vi "Set_Hi-Tec_client.vi"(4 "Gas Line Name":T1, 5 "Row No":i32=1, 6 "Strength (% by volume)":dbl format="%.2f", 7 "Carrier_2 Q (l/min)":dbl=20.0 format="%.2f", 8 "Carrier_1 Q (l/min)":dbl=20.0 format="%.2f", 9 "Mode":enum16{"Control Hi-Tec", "Check Hi-Tec Demands"}(ring)) -> (0 "error out":errorcluster, 1 "Flowrates (kg/min)":dbl[](array[numeric]) format="%.4f")   [LabVIEW 2022 SP3]
doc: "This is an example of using features of the VI Server as a client. It shows how you might browse from one or more applications that may be exporting data from one or more data stations. \n\nThe example shows how to query a server for its list of exported VIs, how to get references to the VIs, and how call them with the Call By Reference function."
uses:
  Anemometry/Anemometry Sub Vis/Controls/GMU Gas Line Name.ctl
  Anemometry/Anemometry Sub Vis/Globals/Preference_global.vi
panel:
  out "Iterations":i32
  in  "Server type":refnum<vi>
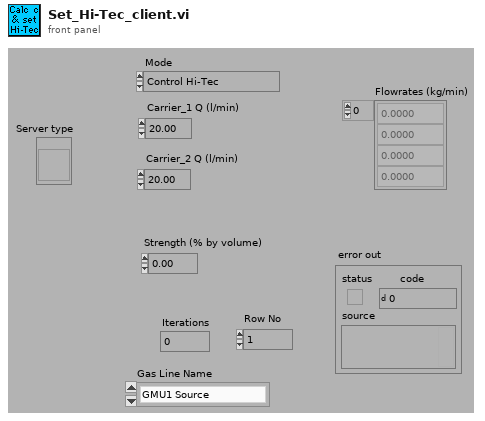
[diagram p1: front panel]
types:
  T1 = typedef "GMU Gas Line Name.ctl" = enum16{"GMU1 Source", "GMU2 Source", "GMU2 Calib", "CPP GRC-A", "CPP GRC-B"}
  T2 = typedef "Server_Comms.ctl" = enum16{"Do Not Link To Server", "Server Link Healthy"}
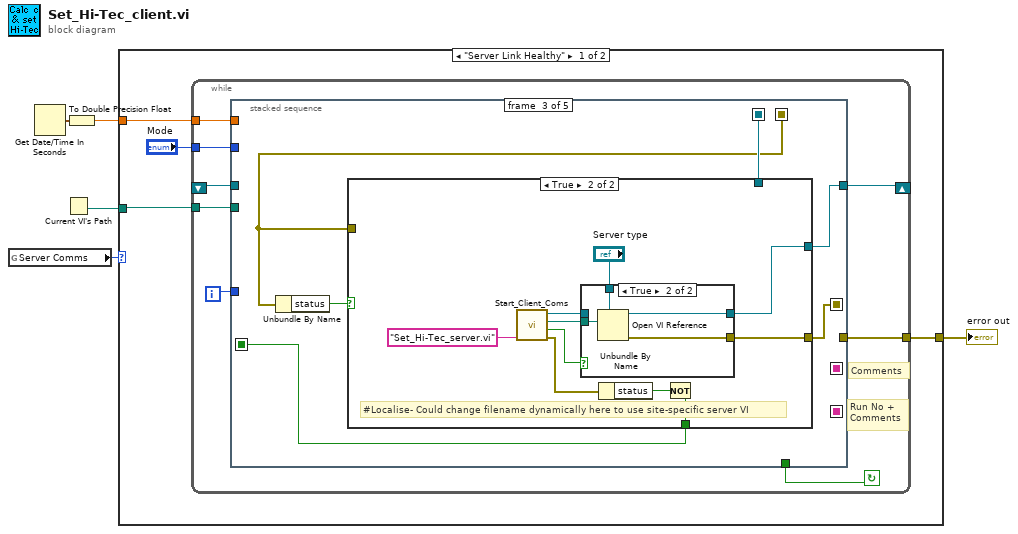
[diagram p0: block diagram]
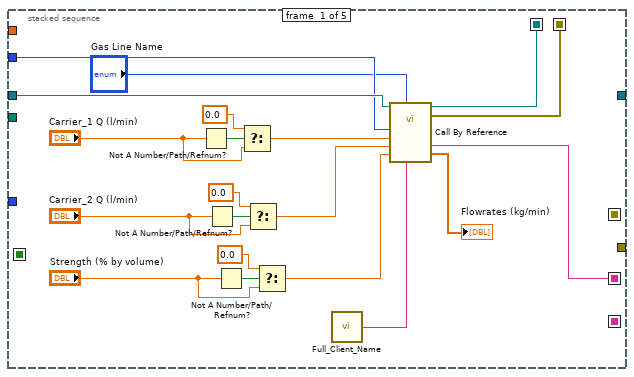
[diagram p2: hidden frame]
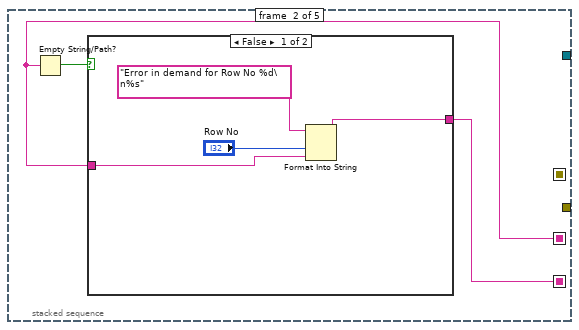
[diagram p3: hidden frame]
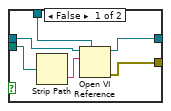
[diagram p6: hidden frame]
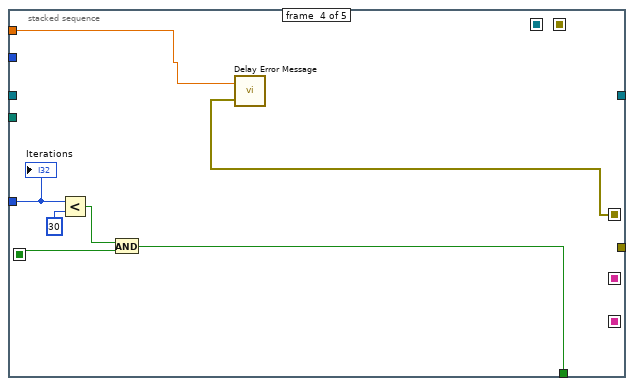
[diagram p7: hidden frame]
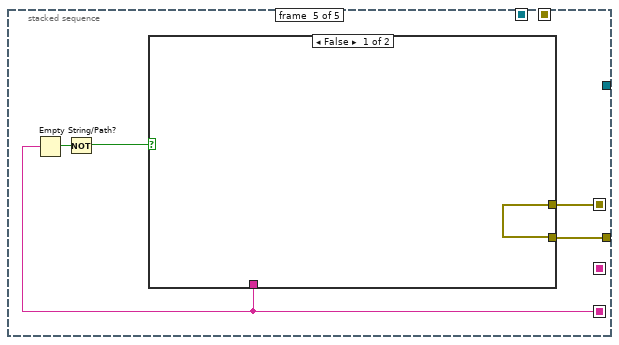
[diagram p8: hidden frame]
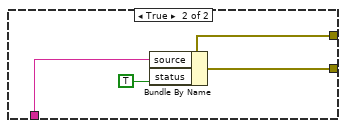
[diagram p9: hidden frame]
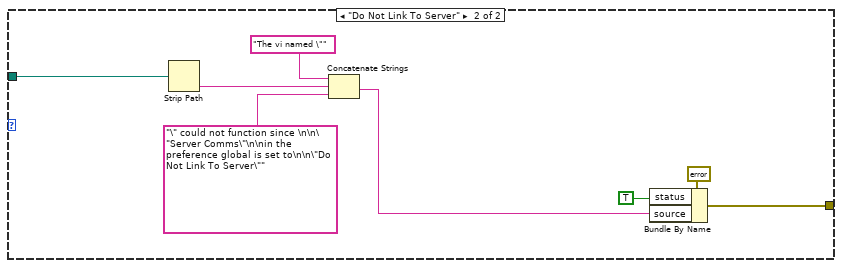
[diagram p10: hidden frame]
diagram:
  n1 = global read "Preference_global.vi" "Server Comms"() -> (w5:T2)
  n2 = Get Date/Time In Seconds() -> (seconds since 1Jan1904=w2:timestamp)
  n3 = Current VI's Path() -> (path=w4:path)
  n4 = To Double Precision Float(number=w2) -> (double precision float=w1:dbl)
  n5 = case shown="\"Server Link Healthy\"" w5 {
    tunnel: [w9 w93] -> w3
    tunnel: w4 -> [w7 w92]
    tunnel: w1 -> [w6 _]
    frame "Server Link Healthy" {
      n6 = while {
        tunnel: w7 -> [w11]
        tunnel: "Mode" -> [w12]
        tunnel: [w13] -> w9
        shift-left: _ -> [w17]
        shift-right: [w16] -> _
        tunnel: w6 -> [w10]
        i -> [w15]
        stop <- w14 continue-if-true
        # "Run No +\nComments"
        # "Comments"
        n7 = stacked-sequence {
          seq-local: [w36 _ _ _ _] -> [_ _ w51 _ _]
          seq-local: [w35 _ _ _ _] -> [_ _ w48 _ _]
          seq-local: [_ _ w46 _ _] -> [_ _ _ w78 _]
          seq-local: [w33 _ _ _ _] -> [_ w39 _ _ _]
          seq-local: [_ w38 _ _ _] -> [_ _ _ _ w84]
          seq-local: [_ _ w47 _ _] -> [_ _ _ w75 w86]
          tunnel: w17 -> [w37 _ _ _ _]
          tunnel: [_ _ w50 _ _] -> w16
          tunnel: w15 -> [_ _ _ w81 _]
          tunnel: [_ _ _ w77 _] -> w14
          tunnel: [_ _ _ _ w85] -> w13
          tunnel: w12 -> [w32 _ _ _ _]
          tunnel: w11 -> [_ _ _ _ _]
          tunnel: w10 -> [_ _ _ w76 _]
          frame #0 {
            n8 = Not A Number/Path/Refnum?(number/path/refnum="Carrier_1 Q (l/min)") -> (NaN/Path/Refnum?=w27:bool)
            n9 = Not A Number/Path/Refnum?(number/path/refnum="Carrier_2 Q (l/min)") -> (NaN/Path/Refnum?=w30:bool)
            n10 = Not A Number/Path/Refnum?(number/path/refnum="Strength (% by volume)") -> (NaN/Path/Refnum?=w23:bool)
            n11 = Select(t=0.0, s=w27, f="Carrier_1 Q (l/min)") -> (s? t:f=w21:dbl)
            n12 = Select(t=0.0, s=w30, f="Carrier_2 Q (l/min)") -> (s? t:f=w20:dbl)
            n13 = Select(t=0.0, s=w23, f="Strength (% by volume)") -> (s? t:f=w19:dbl)
            n14 = call "Full_Client_Name.vi"() -> ("Client Name"=w31:string)
            n15 = call-by-ref "?"(reference=w37, "Client Name"=w31, "Gas Line Name"="Gas Line Name", "Strength (% by volume)"=w19, "Carrier_2 Q (l/min)"=w20, "Carrier_1 Q (l/min)"=w21, "Mode"=w32) -> (reference out=w36:refnum<vi>, error out=w35:errorcluster, "Flowrates (kg/min)"=→"Flowrates (kg/min)":dbl[], "Comment"=w33:string)  [unwired: 3 in]
          }
          frame #1 {
            n16 = Empty String/Path?(string/path=w39) -> (empty?=w40:bool)
            n17 = case shown="False" w40 {
              tunnel: w39 -> [w41 w45]
              tunnel: [w43 w45] -> w38
              frame False {
                n18 = Format Into String(format string="Error in demand for Row No %d\n%s" ("Format String"), "Row No", w41) -> (resulting string=w43:string)  [unwired: 2 in, 1 out]
              }
              frame True {
              }
            }
          }
          frame #2 {
            n19 = Unbundle By Name(w48) -> ("status"=w49:bool)
            n20 = case shown="True" w49 {
              selector: w49 -> [w52 _]
              tunnel: w51 -> [w54 _]
              tunnel: [w54 w59] -> w50
              tunnel: [w53 w58] -> w47
              tunnel: w48 -> [w53 _]
              tunnel: [w52 w55] -> w46
              frame False {
              }
              frame True {
                # "#Localise- Could change filename dynamically here to use site-specific server VI"
                n21 = call "Start_Client_Coms.vi"("VI name to run on server"="Set_Hi-Tec_server.vi") -> ("LabVIEW application reference"=w63:refnum<vi>, "Checked VI name"=w64:path, "Local Call"=w62:bool, "Error cluster"=w56:errorcluster)  [unwired: 1 in]
                n22 = case shown="True" w62 {
                  tunnel: "Server type" -> [w66 w73]
                  tunnel: w64 -> [w67 w74]
                  tunnel: w63 -> [w65 _]
                  tunnel: [w69 w72] -> w59
                  tunnel: [w68 w71] -> w58
                  frame False {
                    n23 = Strip Path(path=w67) -> (name=w70:string)  [unwired: 1 out]
                    n24 = Open VI Reference(type specifier VI Refnum (for type only)=w66, application reference (local)=w65, vi path=w70) -> (vi reference=w69:refnum<vi>, error out=w68:errorcluster)  [unwired: 1 in, 2 out]
                  }
                  frame True {
                    n25 = Open VI Reference(type specifier VI Refnum (for type only)=w73, vi path=w74) -> (vi reference=w72:refnum<vi>, error out=w71:errorcluster)  [unwired: 1 in, 3 out]
                  }
                }
                n26 = Unbundle By Name(w56) -> ("status"=w57:bool)
                n27 = Not(x=w57) -> (.not. x?=w55:bool)
              }
            }
          }
          frame #3 {
            n28 = Less?(x=w81, y=30) -> (x < y?=w79:bool)
            n29 = And(x=w79, y=w78) -> (x .and. y?=w77:bool)
            n30 = call "Delay Error Message.vi"("error in (no error)"=w75, "Seconds since 1904"=w76) -> ()  [unwired: 2 in]
            "Iterations" <- w81
          }
          frame #4 {
            n31 = Empty String/Path?(string/path=w84) -> (empty?=w83:bool)
            n32 = Not(x=w83) -> (.not. x?=w82:bool)
            n33 = case shown="False" w82 {
              tunnel: w86 -> [w87 w91]
              tunnel: w84 -> [_ w88]
              tunnel: [w87 w90] -> w85
              frame False {
              }
              frame True {
                n34 = Bundle By Name(cluster=w91, "source"=w88, "status"=TRUE ("Bundle Element")) -> (w90:errorcluster)
              }
            }
          }
        }
      }
    }
    frame "Do Not Link To Server" {
      n35 = Strip Path(path=w92) -> (name=w98:string)  [unwired: 1 out]
      n36 = Concatenate Strings("The vi named \"", w98, "\" could not function since \n\n\"Server Comms\"\n\nin the preference global is set to\n\n\"Do Not Link To Server\"") -> (w95:string)
      n37 = Bundle By Name(cluster=errorcluster {"status"=FALSE, "code"=0, "source"=""}, "status"=TRUE ("Bundle Element"), "source"=w95) -> (w93:errorcluster)
    }
  }
  "error out" <- w3
